vi "Translator.TranslateThis.Exit.vi"(8 "error in":errorcluster) -> (0 "error out":errorcluster)   [LabVIEW 2016]
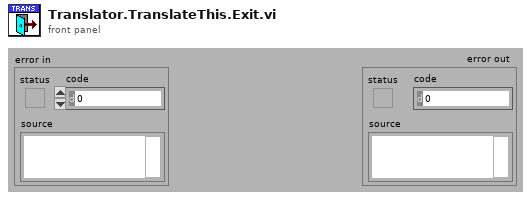
[diagram p1: front panel]
types:
  T1 = enum32{"invalid app kind", "Development System", "Run Time System", "Student Edition", "Embedded LabVIEW", "Evaluation", "Custom"}
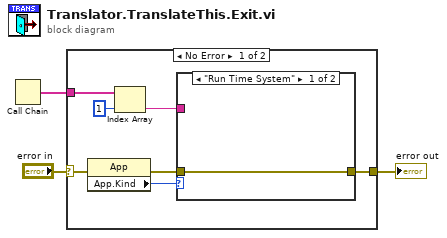
[diagram p0: block diagram]
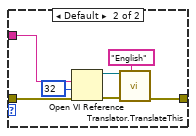
[diagram p2: hidden frame]
diagram:
  n1 = Call Chain() -> (call chain=w1:string[])
  n2 = case shown="No Error" "error in" {
    selector: "error in" -> [w4 w19]
    tunnel: [w10 w19] -> w3
    tunnel: w1 -> [w7 _]
    frame No Error {
      n3 = property class="App"(error in=w4) -> (error out=w9:errorcluster, "App.Kind"=w8:T1)  [unwired: 1 in, 1 out]
      n4 = Index Array(array=w7, index=1) -> (element=w5:string)
      n5 = case shown="\"Run Time System\"" w8 {
        tunnel: [w11 w14] -> w10
        tunnel: w9 -> [w11 w17]
        tunnel: w5 -> [_ w13]
        frame "Run Time System" {
        }
        frame Default {
          n6 = Open VI Reference(vi path=w13, options=32, error in (no error)=w17) -> (vi reference=w15:refnum<vi>, error out=w16:errorcluster)  [unwired: 1 in, 2 out]
          n7 = call "Translator.TranslateThis.vi"("Language (English)"="English" ("Language"), "error in"=w16, "vi reference"=w15) -> ("error out"=w14:errorcluster)  [unwired: 8 in]
        }
      }
    }
    frame Error {
    }
  }
  "error out" <- w3
